vi "writeByteInstruction.vi"(8 "error in (no error)":errorcluster, 10 "Input":u8, 11 "ModbusBuffer in":refnum<class "ModbusBuffer.lvclass">) -> (0 "error out":errorcluster, 2 "Output":u16, 3 "ModbusBuffer out":refnum<class "ModbusBuffer.lvclass">)   [LabVIEW 2016, in "RTModbus.lvlib" / "ModbusBuffer.lvclass"]
uses:
  ModbusBuffer.lvclass
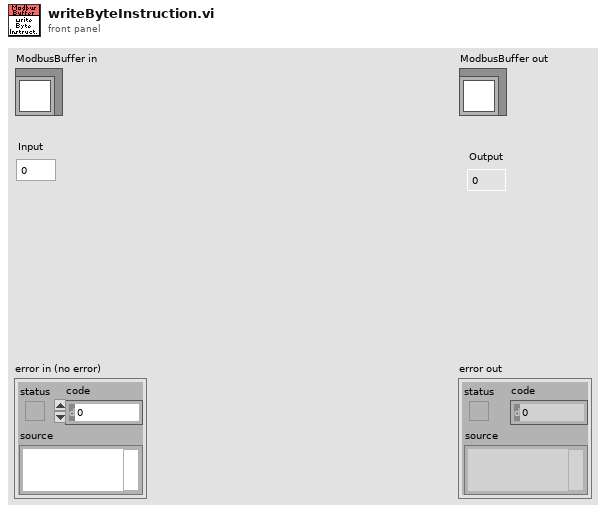
[diagram p1: front panel]
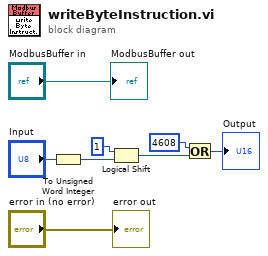
[diagram p0: block diagram]
diagram:
  n1 = To Unsigned Word Integer(number="Input") -> (unsigned 16bit integer=w3:u16)
  n2 = Logical Shift(y=i16 1, x=w3) -> (x << y=w5:u16)
  n3 = Or(x=u16 4608, y=w5) -> (x .or. y?=→"Output":u16)
  "error out" <- "error in (no error)"
  "ModbusBuffer out" <- "ModbusBuffer in"
